vi "Move GULP Files to Buckets.vi"() -> ()   [LabVIEW 2010]
panel:
  in  "# per bucket":i32
  in  "GULP Files Directory":path
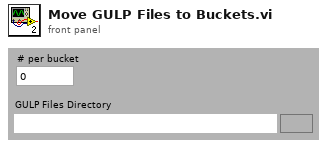
[diagram p1: front panel]
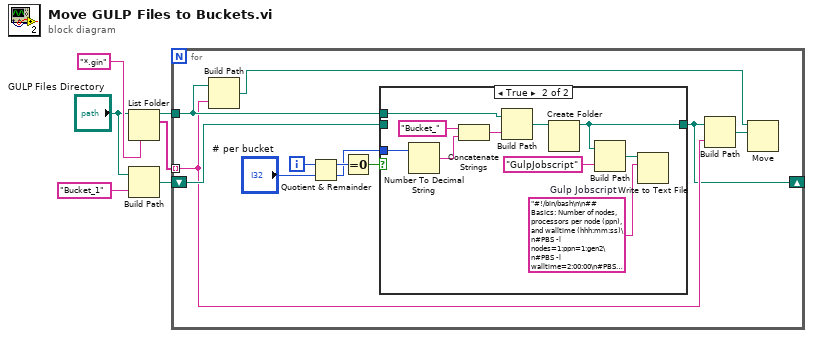
[diagram p0: block diagram]
diagram:
  n1 = List Folder(path="GULP Files Directory", pattern="*.gin") -> (path out=w4:path, filenames=w5:string[])  [unwired: 2 in, 2 out]
  n2 = Build Path(base path="GULP Files Directory", name or relative path="Bucket_1") -> (appended path=w1:path)
  n3 = for {
    tunnel: w5 -> [w9] mode=indexing
    tunnel: w4 -> [w11]
    shift-right: [w7] -> _
    shift-left: w1 -> [w14]
    i -> [w17]
    n4 = Build Path(base path=w11, name or relative path=w9) -> (appended path=w10:path)
    n5 = Quotient & Remainder(x=w17, y="# per bucket") -> (x-y*floor(x/y)=w15:i32, floor(x/y)=w12:i32)
    n6 = Equal To 0?(x=w15) -> (x = 0?=w13:bool)
    n7 = case shown="True" w13 {
      tunnel: w14 -> [w18 _]
      tunnel: [w18 w21] -> w7
      tunnel: w11 -> [_ w27]
      tunnel: w12 -> [_ w25]
      frame False {
      }
      frame True {
        w22 = "#!/bin/bash\n\n##  Basics: Number of nodes, processors per node (ppn), and walltime (hhh:mm:ss)\n#PBS -l nodes=1:ppn=1:gen2\n#PBS -l walltime=2:00:00\n#PBS -N GulpCalc\n#PBS -A cnm35383 # Robert Klie \n\n## File names for stdout and stderr.  If not set here, the defaults\n## are <JOBNAME>.o<JOBNUM> and <JOBNAME>.e<JOBNUM>\n#PBS -o gulp.out\n#PBS -e err.out\n\n## send mail at begin, end, abort, or never (b, e, a, n)\n#PBS -m bea\n# change into the directory where qsub will be executed\ncd $PBS_O_WORKDIR\n\n# count allocated cores\nNPROCS=`wc -l < $PBS_NODEFILE`\n\n# start MPI job over default interconnect\n     for i in $( ls | grep .gin)\ndo\noutputname=$i\".out\"\ngulp < $i > $outputname\n##mpirun -machinefile $PBS_NODEFILE -np $NPROCS gulp < $i > $outputname\n##echo Submitting $i\ndone"  # Gulp Jobscript
        n8 = Number To Decimal String(number=w25) -> (decimal integer string=w24:string)  [unwired: 1 in]
        n9 = Concatenate Strings("Bucket_" ("string"), w24) -> (w23:string)
        n10 = Build Path(base path=w27, name or relative path=w23) -> (appended path=w28:path)
        n11 = Create Folder(path (use dialog)=w28) -> (created path=w21:path)  [unwired: 2 in, 2 out]
        n12 = Build Path(base path=w21, name or relative path="GulpJobscript") -> (appended path=w20:path)
        n13 = Write to Text File(file (use dialog)=w20, text=w22) -> ()  [unwired: 2 in, 3 out]
      }
    }
    n14 = Build Path(base path=w7, name or relative path=w9) -> (appended path=w8:path)
    n15 = Move(source path=w10, 10:w8) -> ()  [unwired: 3 in, 3 out]
  }
